vi "FRCts20_Backend_Test_Event_GETFiltered.vi"(8 "error in (no error)":errorcluster, 11 "Name":string) -> (0 "error out":errorcluster, 1 "Time (ms)":u32, 2 "Status":string, 3 "Event Out":T2, 5 "Success":bool)   [LabVIEW 2014, in "FRCts20_Backend_TestCode.lvlib"]
uses:
  FRCts20_Backend_TestCode.lvlib
  FRCts20_Backend_API/FRCts20_Backend_API_Event.ctl
  FRCts20_Backend_API/FRCts20_Backend_API_SW.ctl
  FRCts20_Backend_API/FRCts20_Backend_API_Command_Event.ctl
  FRCts20_Backend_API/FRCts20_Backend_API_Event.vi
  FRCts20_Backend_API/FRCts20_Backend_API.lvlib
panel:
  in  "SWType":T1
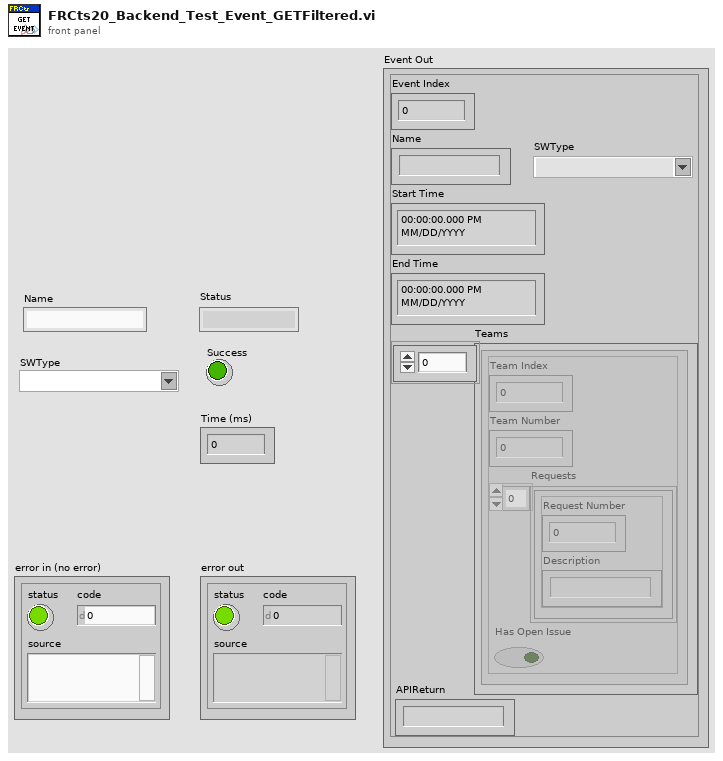
[diagram p1: front panel]
types:
  T1 = typedef "FRCts20_Backend_API.lvlib/FRCts20_Backend_API_SW.ctl" = string
  T2 = typedef "FRCts20_Backend_API.lvlib/FRCts20_Backend_API_Event.ctl" = cluster{"Event Index":u32, "Name":string, "Start Time":timestamp, "End Time":timestamp, "Teams":cluster{"Team Index":u32, "Team Number":u32, "Requests":cluster{"Request Number":u32, "Description":string}[], "Has Open Issue":bool}[], "SWType":T1, "APIReturn":string}
  T3 = typedef "FRCts20_Backend_API.lvlib/FRCts20_Backend_API_Command_Event.ctl" = string
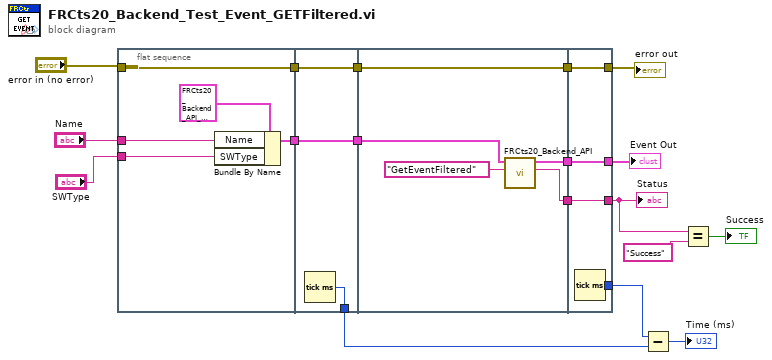
[diagram p0: block diagram]
diagram:
  n1 = flat-sequence {
    tunnel: "error in (no error)" -> [w23]
    tunnel: [w23] -> w16
    tunnel: [w21] -> w3
    tunnel: "Name" -> [w20]
    tunnel: "SWType" -> [w19]
    tunnel: [w26] -> w9
    tunnel: [w25] -> w15
    tunnel: w16 -> [w25]
    tunnel: [w24] -> w4
    tunnel: w3 -> [w24]
    tunnel: [w31] -> w14
    tunnel: w15 -> [w31]
    tunnel: [w30] -> w8
    tunnel: [w29] -> w6
    tunnel: w4 -> [w28]
    tunnel: [w35] -> w10
    tunnel: [w34] -> w12
    tunnel: w14 -> [w34]
    tunnel: [w33] -> w7
    tunnel: w8 -> [w33]
    tunnel: [w32] -> w5
    tunnel: w6 -> [w32]
    frame #0 {
      n2 = Bundle By Name(cluster=T2 {"Event Index"=0, "Name"="", "Start Time"=timestamp(0 s since 1904-01-01), "End Time"=timestamp(0 s since 1904-01-01), "Teams"=[], "SWType"="", "APIReturn"=""} ("Event In"), "Name"=w20, "SWType"=w19) -> (w21:T2)
    }
    frame #1 {
      n3 = Tick Count (ms)() -> (millisecond timer value=w26:u32)
    }
    frame #2 {
      n4 = call-poly "FRCts20_Backend_API.vi"("Command"=T3 "GetEventFiltered", "Event In"=w28) -> ("Status"=w29:string, "Event Out"=w30:T2)  [unwired: 7 in, 1 out]
    }
    frame #3 {
      n5 = Tick Count (ms)() -> (millisecond timer value=w35:u32)
    }
  }
  n6 = Subtract(x=w10, y=w9) -> (x-y=→"Time (ms)":u32)
  n7 = Equal?(x=w5, y="Success") -> (x = y?=→"Success":bool)
  "Event Out" <- w7
  "Status" <- w5
  "error out" <- w12
